vi "read_check_value.vi"(0 "Array values":dbl[](array[numeric])) -> (1 "Pressure":dbl, 2 "Knob_voltage":dbl, 3 "Temparature":dbl, 4 "Error thermometer?":bool, 6 "Error pressure?":bool, 8 "Voltage":dbl, 10 "Error voltage?":bool, 12 "Cluster of values":cluster{dbl, dbl, dbl, dbl}, 13 "Error amperage?":bool, 14 "Amperage":dbl)   [LabVIEW 2015]
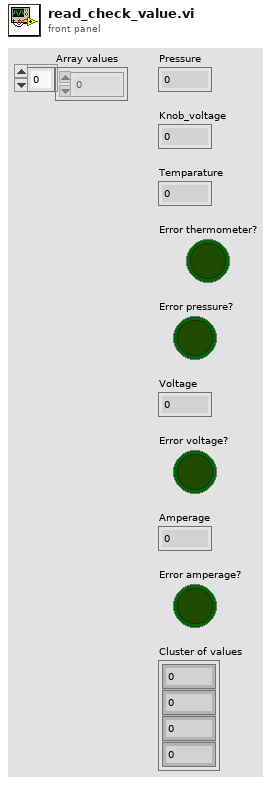
[diagram p1: front panel]
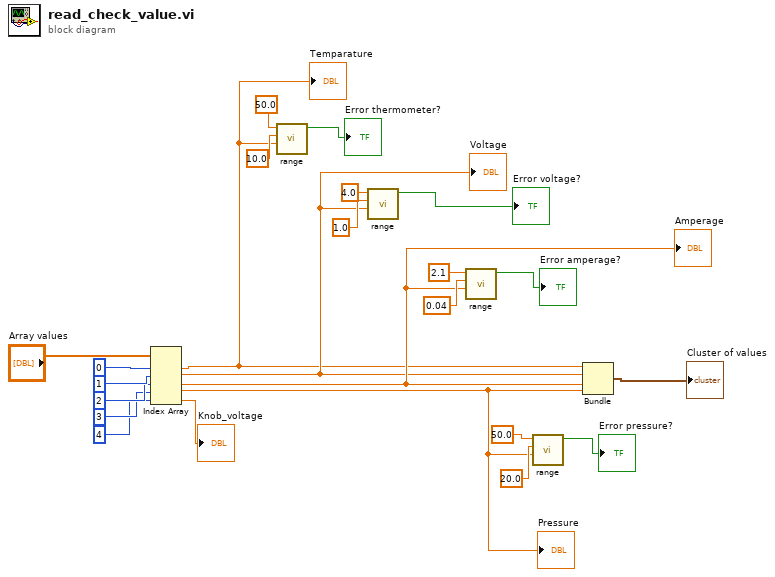
[diagram p0: block diagram]
diagram:
  n1 = Index Array(array="Array values", index #1=0 ("index"), index #2=1 ("index"), index #3=2 ("index"), index #4=3 ("index"), index #5=4 ("index")) -> (element #1=w10:dbl, element #2=w12:dbl, element #3=w17:dbl, element #4=w21:dbl, element #5=→"Knob_voltage":dbl)
  "Temparature" <- w10
  "Voltage" <- w12
  "Amperage" <- w17
  "Pressure" <- w21
  n2 = call "range.vi"("Value"=w10, "lower limit"=10.0, "upper limit"=50.0) -> ("In range?"=→"Error thermometer?":bool)  [unwired: 8 in]
  n3 = call "range.vi"("Value"=w12, "lower limit"=1.0, "upper limit"=4.0) -> ("In range?"=→"Error voltage?":bool)  [unwired: 8 in]
  n4 = call "range.vi"("Value"=w17, "lower limit"=0.04, "upper limit"=2.1) -> ("In range?"=→"Error amperage?":bool)  [unwired: 8 in]
  n5 = call "range.vi"("Value"=w21, "lower limit"=20.0, "upper limit"=50.0) -> ("In range?"=→"Error pressure?":bool)  [unwired: 8 in]
  n6 = Bundle(w10, w12, w17, w21) -> (→"Cluster of values":cluster{dbl, dbl, dbl, dbl})  [unwired: 1 out]
